vi "Display Image.vi"(7 "Factor":dbl=1.0, 8 "error in (no error)":errorcluster, 9 "Brightness":u8=50 max=100 step=1, 10 "path to BMP file on myRio local filesystem":path=path "/home/admin/images/test.bmp", 11 "Refnum in":refnum<k20>) -> (0 "error out":errorcluster, 3 "Refnum out":refnum<k20>, 4 "Rectangle":T1, 5 "LED Matrix":picture, 6 "image depth":i32)   [LabVIEW 2013]
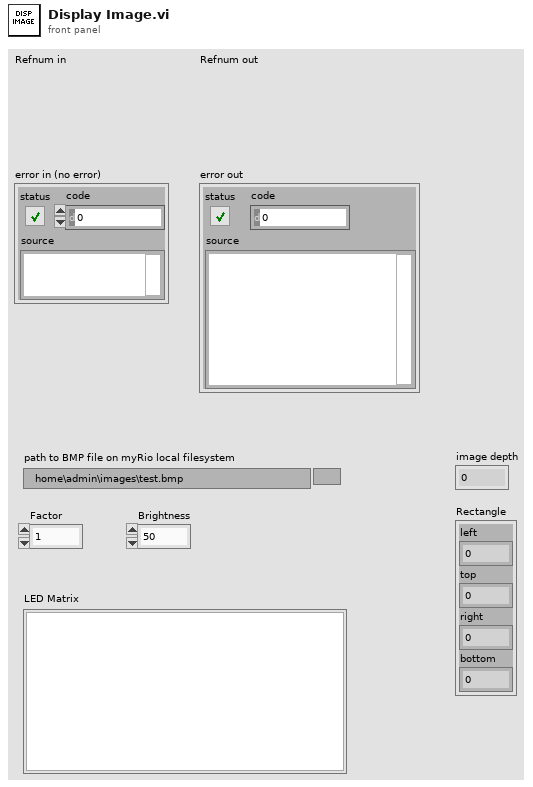
[diagram p1: front panel]
types:
  T1 = cluster{"left":i16, "top":i16, "right":i16, "bottom":i16}
  T2 = typedef "imagedata.ctl" = cluster{"image type":i32, "image depth":i32, "image":u8[], "mask":u8[], "colors":u32[], "Rectangle":cluster{"left":i16, "top":i16, "right":i16, "bottom":i16}}
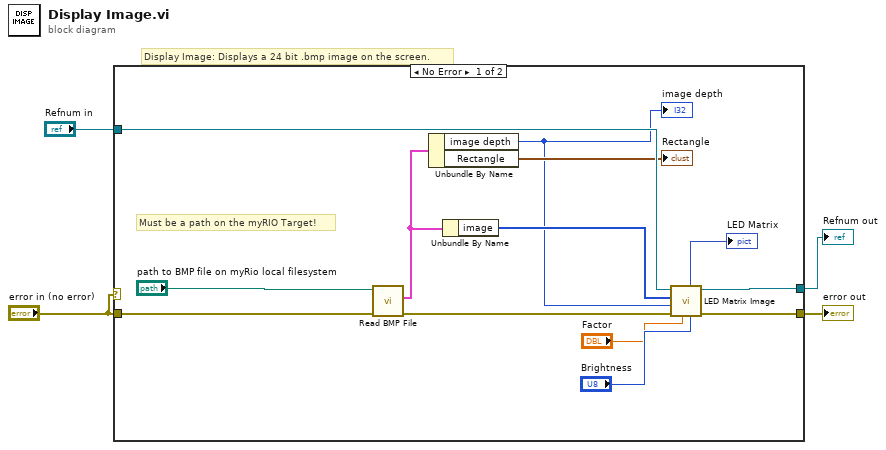
[diagram p0: block diagram]
diagram:
  # "Display Image: Displays a 24 bit .bmp image on the screen."
  n1 = case shown="No Error" "error in (no error)" {
    tunnel: "error in (no error)" -> [w17 w18]
    tunnel: "Refnum in" -> [w13 w19]
    tunnel: [w16 w18] -> w3
    tunnel: [w15 w19] -> w2
    frame No Error {
      # "Must be a path on the myRIO Target!"
      n2 = call <vilib>:"Read BMP File.vi"("error in (no error)"=w17, "path to BMP file"="path to BMP file on myRio local filesystem") -> ("error out"=w12:errorcluster, "image data"=w11:T2)  [unwired: 7 in, 1 out]
      n3 = Unbundle By Name(w11) -> ("image depth"=w5:i32, "Rectangle"=→"Rectangle":T1)
      "image depth" <- w5
      n4 = Unbundle By Name(w11) -> ("image"=w9:u8[])
      n5 = call "LED Matrix Image.vi"("Brightness"="Brightness", "Factor"="Factor", "error in (no error)"=w12, "image depth"=w5, "image"=w9, "Refnum in"=w13) -> ("error out"=w16:errorcluster, "Refnum out"=w15:refnum<k20>, "LED Matrix"=→"LED Matrix":picture)  [unwired: 3 in]
    }
    frame Error {
    }
  }
  "error out" <- w3
  "Refnum out" <- w2
